vi "VarMessage Probe.vi"(1 "Message":refnum<class "VarMessage.lvclass">) -> (0 "Boolean":bool)   [LabVIEW 2011, in "Messenging.lvlib" / "VarMessage.lvclass"]
uses:
  VarMessage.lvclass
  TextVarientMessage/MSG.lvclass
panel:
  out "Label 2":string
  out "Label":string caption="Label (or Data Name)"
  out "Varient":variant
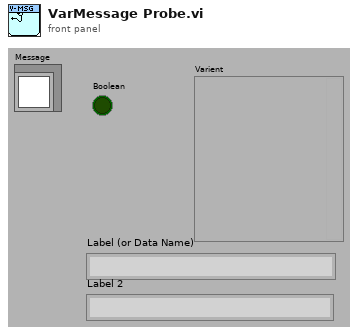
[diagram p1: front panel]
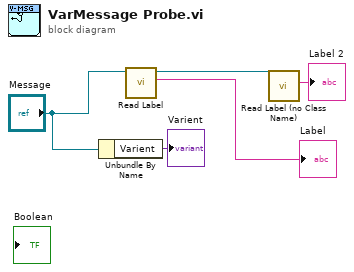
[diagram p0: block diagram]
diagram:
  n1 = Unbundle By Name("Message") -> ("Varient"=→"Varient":variant)
  n2 = call-dynamic "Read Label.vi"("Message"="Message") -> ("Label"=→"Label":string, "Message"=w2:refnum<class "VarMessage.lvclass">)  [unwired: 1 in, 8 out]
  n3 = call "Read Label (no Class Name).vi"("MSG.lvclass in"=w2) -> ("Label"=→"Label 2":string)  [unwired: 10 out]
